vi "Write to lifter config.vi"(0 "Insert name":enum16{"Insert #1", "Insert #2", "CALIB_INSERT"}(ring), 1 "Default":bool, 5 "File Name":string="Lifter config", 7 "Bottom":dbl format="%#_3g", 9 "Middle":dbl, 11 "Top":dbl, 12 "error in (no error)":errorcluster) -> (4 "Cup locations":dbl[](array[numeric]), 15 "error out":errorcluster)   [LabVIEW 2019]
uses:
  <vilib>/Utility/config.llb/Write Key (Double).vi
  <vilib>/Utility/config.llb/NI_LVConfig.lvlib
panel:
  out "appended path":path
  out "concatenated string":string
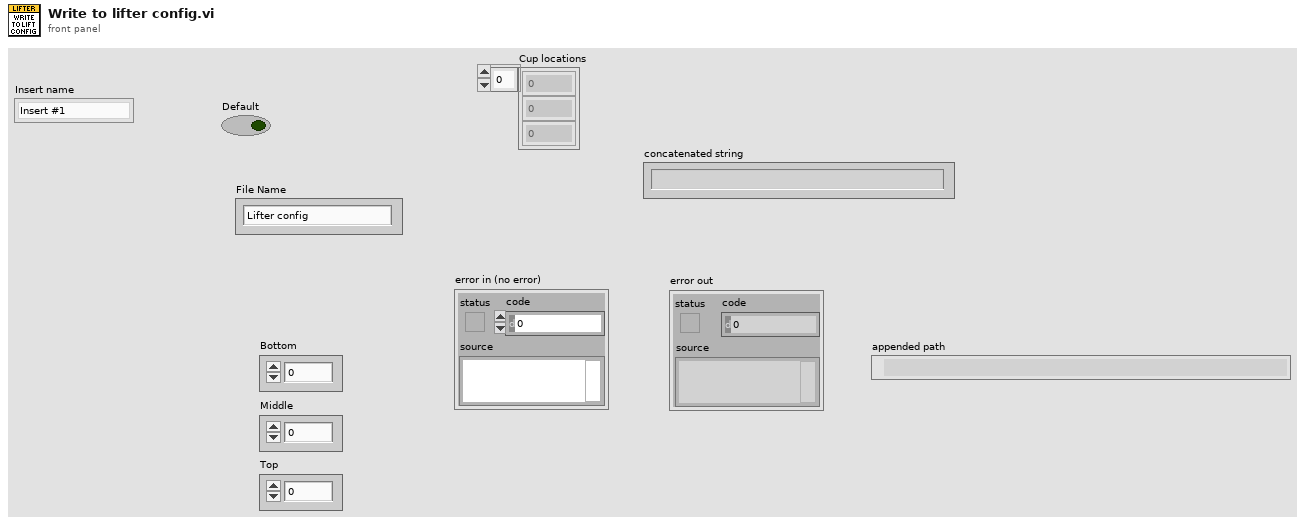
[diagram p1: front panel]
types:
  T1 = typedef "NI_LVConfig.lvlib/Config Data RefNum.ctl" = refnum<k1>
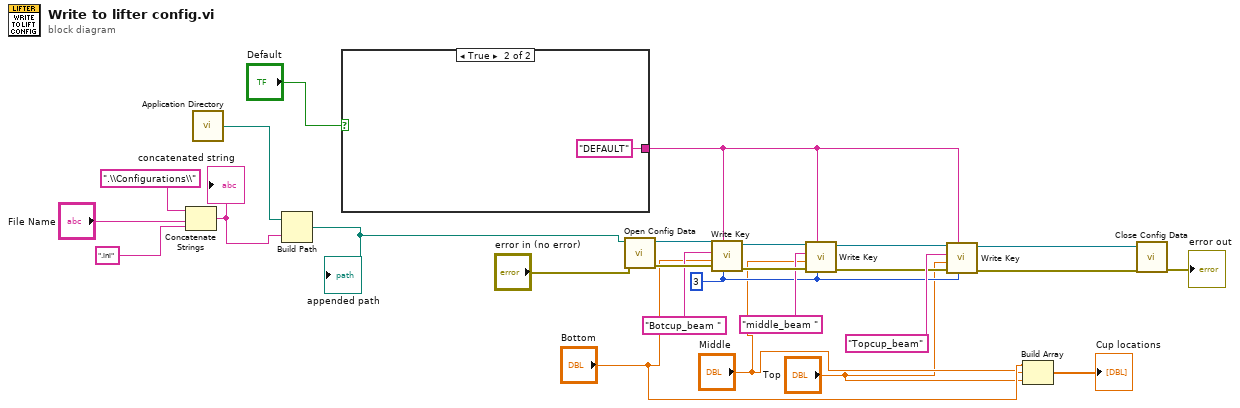
[diagram p0: block diagram]
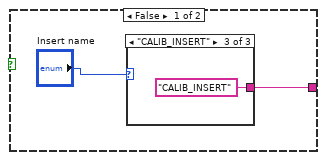
[diagram p2: hidden frame]
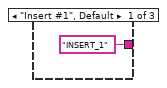
[diagram p3: hidden frame]
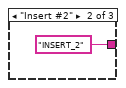
[diagram p4: hidden frame]
diagram:
  w7 = i16 3 ("precision (6)")
  n1 = Concatenate Strings(".\\Configurations\\" ("string"), "File Name", ".ini" ("string")) -> (w18:string)
  "concatenated string" <- w18
  n2 = call <vilib>:"Application Directory.vi"() -> ("Application Directory"=w16:path)
  n3 = Build Path(base path=w16, name or relative path=w18) -> (appended path=w13:path)
  "appended path" <- w13
  n4 = case shown="True" "Default" {
    tunnel: [w27 "DEFAULT" ("section")] -> w6
    frame False {
      n5 = case shown="\"CALIB_INSERT\"" "Insert name" {
        tunnel: ["INSERT_1" ("section") "INSERT_2" ("section") "CALIB_INSERT" ("section")] -> w27
        frame "Insert #1", Default {
        }
        frame "Insert #2" {
        }
        frame "CALIB_INSERT" {
        }
      }
    }
    frame True {
    }
  }
  n6 = call <vilib>:"Open Config Data.vi"("error in (no error)"="error in (no error)", "configuration file path"=w13) -> ("error out"=w23:errorcluster, "refnum"=w26:T1)  [unwired: 7 in, 1 out]
  n7 = call-poly <vilib>:"Write Key.vi"("precision (6)"=w7, "section"=w6, "error in (no error)"=w23, "value"="Bottom", "key"="Botcup_beam ", "refnum"=w26) -> ("error out"=w24:errorcluster, "refnum out"=w25:T1)  [unwired: 3 in, 1 out]
  n8 = call-poly <vilib>:"Write Key.vi"("precision (6)"=w7, "section"=w6, "error in (no error)"=w24, "value"="Middle", "key"="middle_beam ", "refnum"=w25) -> ("error out"=w11:errorcluster, "refnum out"=w10:T1)  [unwired: 3 in, 1 out]
  n9 = call-poly <vilib>:"Write Key.vi"("precision (6)"=w7, "section"=w6, "error in (no error)"=w11, "value"="Top", "key"="Topcup_beam", "refnum"=w10) -> ("error out"=w9:errorcluster, "refnum out"=w8:T1)  [unwired: 3 in, 1 out]
  n10 = Build Array("Bottom", "Middle", "Top") -> (→"Cup locations":dbl[])
  n11 = call <vilib>:"Close Config Data.vi"("error in (no error)"=w9, "refnum"=w8) -> ("error out"=→"error out":errorcluster)  [unwired: 8 in, 1 out]
